vi "Root Directory Path Global Variable.vi"() -> ()   [LabVIEW 2011]
panel:
  in  "Root Directory Path":path
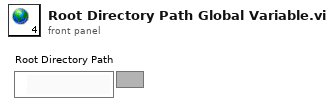
[diagram p1: front panel]
diagram:
